vi "Get DIP State.vi"(0 "error in":errorcluster) -> (1 "DIP State":u32, 2 "error out":errorcluster)   [LabVIEW 2016]
uses:
  Refname/Sensors.ctl
  Refname/Refname to String (Sensors).vi
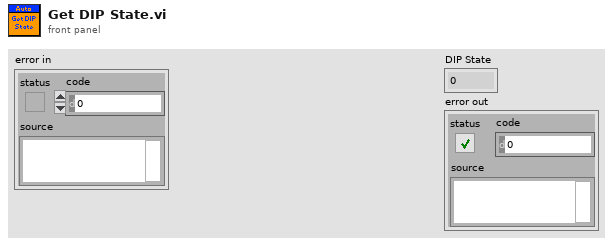
[diagram p1: front panel]
types:
  T1 = typedef "Sensors.ctl" = enum16{"DIP 1", "DIP 2", "DIP 3", "DIP 4", "IMU", "HuskieBoard"}
  T2 = typedef "WPI_SwitchDevRef.ctl" = cluster{"DevStatus":errorcluster, "DIO Channel":T3, "CntIndex":T4, "Normally Closed":bool}
  T3 = typedef "FPGA_DIOChannel.ctl" = enum8{"DIO 0", "DIO 1", "DIO 2", "DIO 3", "DIO 4", "DIO 5", "DIO 6", "DIO 7", "DIO 8", "DIO 9", "DIO MXP 0", "DIO MXP 1", "DIO MXP 2", "DIO MXP 3", "DIO MXP 4", "DIO MXP 5", "DIO MXP 6", "DIO MXP 7", "DIO MXP 8", "DIO MXP 9", "DIO MXP 10", "DIO MXP 11", "DIO MXP 12", "DIO MXP 13", "DIO MXP 14", "DIO MXP 15", "SPI Port CS1", "SPI Port CS2", "SPI Port CS3", "SPI Port MISO", "SPI Port MOSI", "Invalid"}
  T4 = typedef "FPGA_CounterCtrSystemIndex.ctl" = enum8{"Ctr 0", "Ctr 1", "Ctr 2", "Ctr 3", "Ctr 4", "Ctr 5", "Ctr 6", "Ctr 7", "Invalid"}
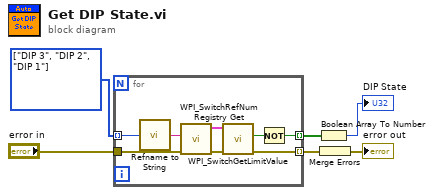
[diagram p0: block diagram]
diagram:
  w4 = T1[] [enum."DIP 3", enum."DIP 2", enum."DIP 1"] items=["DIP 1", "DIP 2", "DIP 3", "DIP 4", "IMU", "HuskieBoard"]
  n1 = for {
    tunnel: w4 -> [w13] mode=indexing
    tunnel: [w14] -> w5 mode=indexing
    tunnel: "error in" -> [w11]
    tunnel: [w8] -> w2 mode=indexing
    n2 = call-poly "Refname to String.vi"("Enum"=w13) -> ("String"=w12:string)
    n3 = call <vilib>:"WPI_SwitchRefNum Registry Get.vi"("error in (no error)"=w11, "refnum name"=w12) -> ("error out"=w9:errorcluster, "SwitchDevRef"=w10:T2)  [unwired: 8 in]
    n4 = call <vilib>:"WPI_SwitchGetLimitValue.vi"("error in (no error)"=w9, "SwitchDevRef"=w10) -> ("error out"=w8:errorcluster, "Switch Pressed"=w7:bool)  [unwired: 7 in, 1 out]
    n5 = Not(x=w7) -> (.not. x?=w14:bool)
  }
  n6 = Boolean Array To Number(Boolean array=w5) -> (number=→"DIP State":u32)
  n7 = Merge Errors(w2) -> (→"error out":errorcluster)
